vi "Read Config.vi"(8 "error in (no error)":errorcluster, 10 "Resource In":variant, 11 "Analyze Parameter Energy in":refnum<class "Analyze Parameter Energy.lvclass">) -> (0 "error out":errorcluster, 2 "Resource Out":variant, 3 "Analyze Parameter Energy out":refnum<class "Analyze Parameter Energy.lvclass">)   [LabVIEW 2020, in "Analyze Parameter Energy.lvclass"]
uses:
  Analyze Parameter Energy.lvclass
  C:/POLARIS Programme/POLARIS-AS-3-Cams/Submodules/HIJ Vision/Analyze/Analyze Parameter/Analyze Parameter Base/Analyze Parameter Base.lvclass
  <vilib>/Utility/config.llb/Config Data RefNum.ctl
  Analyze Parameter Energy.lvclass/Analyze Parameter Energy.ctl
  <vilib>/Utility/config.llb/Read Key (Double).vi
  <vilib>/Utility/config.llb/NI_LVConfig.lvlib
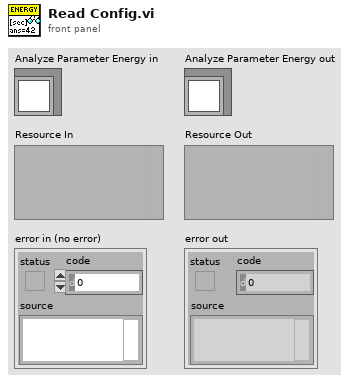
[diagram p1: front panel]
types:
  T1 = typedef "NI_LVConfig.lvlib/Config Data RefNum.ctl" = refnum<k1>
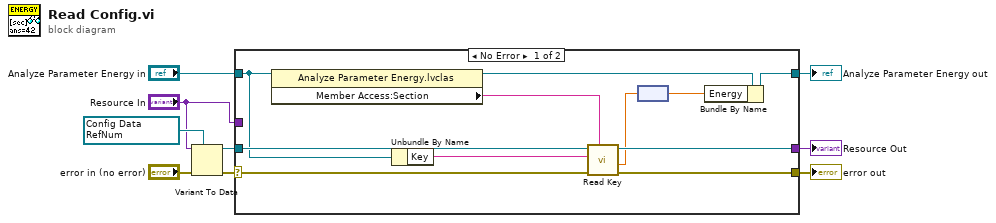
[diagram p0: block diagram]
diagram:
  w8 = T1 refnum items=["config data"] ("refnum")
  n1 = Variant To Data(error in="error in (no error)", type=w8, Variant="Resource In") -> (data=w5:T1, error out=w6:errorcluster)
  n2 = case shown="No Error" w6 {
    selector: w6 -> [w11 w22]
    tunnel: w5 -> [w20 _]
    tunnel: "Analyze Parameter Energy in" -> [w12 w21]
    tunnel: [w16 w21] -> w3
    tunnel: [w18 w23] -> w1
    tunnel: [w10 w22] -> w2
    tunnel: "Resource In" -> [_ w23]
    frame No Error {
      n3 = property class="Analyze Parameter Energy.lvclas"(reference=w12) -> (reference out=w13:refnum<class "Analyze Parameter Energy.lvclass">, "Member Access:Section"=w19:string)  [unwired: 1 in, 1 out]
      n4 = Unbundle By Name(w12) -> ("Key"=w15:string)
      n5 = call-poly <vilib>:"Read Key.vi"("section"=w19, "error in (no error)"=w11, "key"=w15, "refnum"=w20) -> ("error out"=w10:errorcluster, "value"=w17:dbl, "refnum out"=w18:T1)  [unwired: 4 in, 1 out]
      n6 = node(w17) -> (w14:dbl[unit])
      n7 = Bundle By Name(cluster=w13, "Energy"=w14) -> (w16:refnum<class "Analyze Parameter Energy.lvclass">)
    }
    frame Error {
    }
  }
  "error out" <- w2
  "Analyze Parameter Energy out" <- w3
  "Resource Out" <- w1
